vi "ASC字符串至U8数组转换.vi"(11 "ASC字符串":string) -> (3 "U8数组":u8[](array[numeric]))   [LabVIEW 2010]
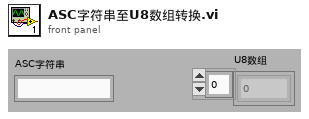
[diagram p1: front panel]
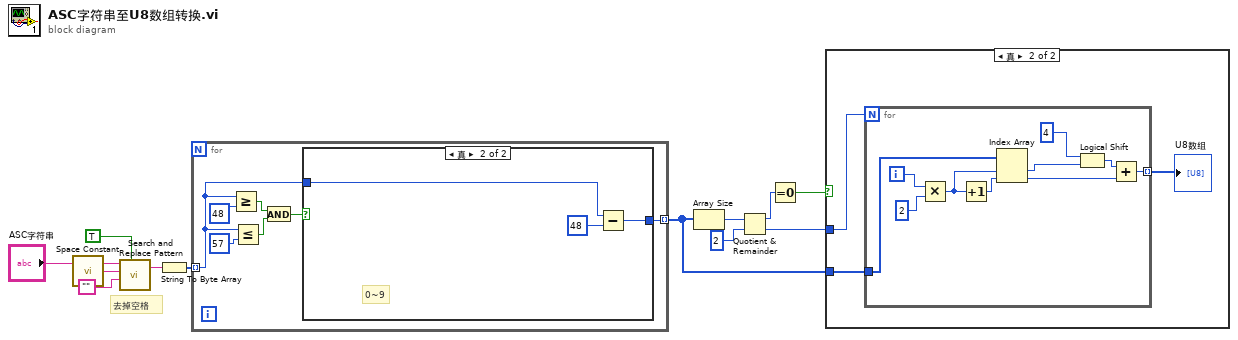
[diagram p0: block diagram]
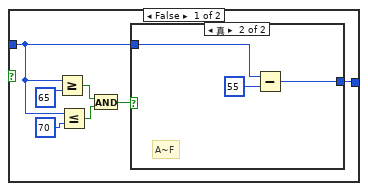
[diagram p3: hidden frame]
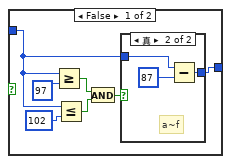
[diagram p4: hidden frame]
diagram:
  # "去掉空格"
  n1 = call <vilib>:"Space Constant.vi"() -> ("String"=w8:string)
  n2 = call <vilib>:"Search and Replace Pattern.vi"("string"="ASC字符串", "regular expression (\"\")"=w8, "replace string (\"\")"="", "replace all? (F)"=TRUE) -> ("result string"=w9:string)  [unwired: 1 in, 1 out]
  n3 = String To Byte Array(string=w9) -> (unsigned byte array=w12:u8[])
  n4 = for {
    tunnel: w12 -> [w13] mode=indexing
    tunnel: [w14] -> w1 mode=indexing
    n5 = Greater Or Equal?(x=w13, y=u8 48) -> (x >= y?=w16:bool)
    n6 = Less Or Equal?(x=w13, y=u8 57) -> (x <= y?=w15:bool)
    n7 = And(x=w16, y=w15) -> (x .and. y?=w17:bool)
    n8 = case shown="真" w17 {
      tunnel: [w20 w42] -> w14
      tunnel: w13 -> [w21 w41]
      frame False {
        n9 = Greater Or Equal?(x=w21, y=u8 65) -> (x >= y?=w24:bool)
        n10 = Less Or Equal?(x=w21, y=u8 70) -> (x <= y?=w23:bool)
        n11 = And(x=w24, y=w23) -> (x .and. y?=w22:bool)
        n12 = case shown="真" w22 {
          tunnel: w21 -> [w28 w39]
          tunnel: [w27 w38] -> w20
          frame False {
            n13 = Greater Or Equal?(x=w28, y=u8 97) -> (x >= y?=w31:bool)
            n14 = Less Or Equal?(x=w28, y=u8 102) -> (x <= y?=w30:bool)
            n15 = And(x=w31, y=w30) -> (x .and. y?=w29:bool)
            n16 = case shown="真" w29 {
              tunnel: w28 -> [w34 w36]
              tunnel: [w34 w35] -> w27
              frame False {
              }
              frame True {
                # "a~f"
                n17 = Subtract(x=w36, y=u8 87) -> (x-y=w35:u8)
              }
            }
          }
          frame True {
            # "A~F"
            n18 = Subtract(x=w39, y=u8 55) -> (x-y=w38:u8)
          }
        }
      }
      frame True {
        # "0~9"
        n19 = Subtract(x=w41, y=u8 48) -> (x-y=w42:u8)
      }
    }
  }
  n20 = Array Size(array=w1) -> (size(s)=w5:i32)
  n21 = Quotient & Remainder(x=w5, y=2) -> (x-y*floor(x/y)=w3:i32, floor(x/y)=w6:i32)
  n22 = Equal To 0?(x=w3) -> (x = 0?=w4:bool)
  n23 = case shown="真" w4 {
    tunnel: w1 -> [_ w46]
    tunnel: w6 -> [_ w44]
    frame False {
    }
    frame True {
      n24 = for {
        N: w44 -> [_]
        tunnel: w46 -> [w56]
        tunnel: [w52] -> w45 mode=indexing
        i -> [w51]
        n25 = Multiply(x=w51, y=2) -> (x*y=w50:i32)
        n26 = Increment(x=w50) -> (x+1=w55:i32)
        n27 = Index Array(array=w56, index #1=w50, index #2=w55) -> (element #1=w48:u8, element #2=w47:u8)
        n28 = Logical Shift(y=i8 4, x=w48) -> (x << y=w53:u8)
        n29 = Add(x=w53, y=w47) -> (x+y=w52:u8)
      }
      "U8数组" <- w45
    }
  }
